vi "ParseCronExpression.vi"(8 "error in (no error)":errorcluster, 9 "values end":u32=59, 10 "values start":u32, 11 "expression":string="2, 45, 2-9,* /15") -> (0 "error out":errorcluster, 3 "comparisons":T1[](array[typedef]))   [LabVIEW 2017, in "CronScheduler.lvlib"]
uses:
  <vilib>/addons/InsightCM/Utilities/CronScheduler/CronScheduler.lvlib
  <vilib>/addons/InsightCM/Utilities/CronScheduler/controls/Compare.ctl
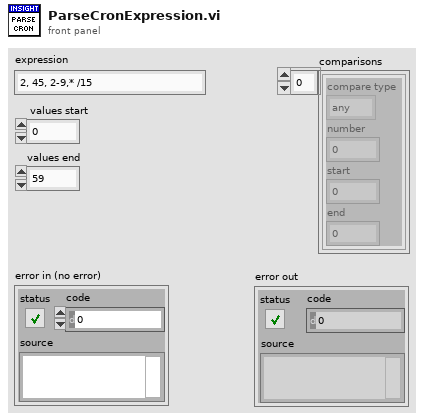
[diagram p1: front panel]
types:
  T1 = typedef "CronScheduler.lvlib/Compare.ctl" = cluster{"compare type":enum16{"any", "number", "range"}, "number":u32, "start":u32, "end":u32}
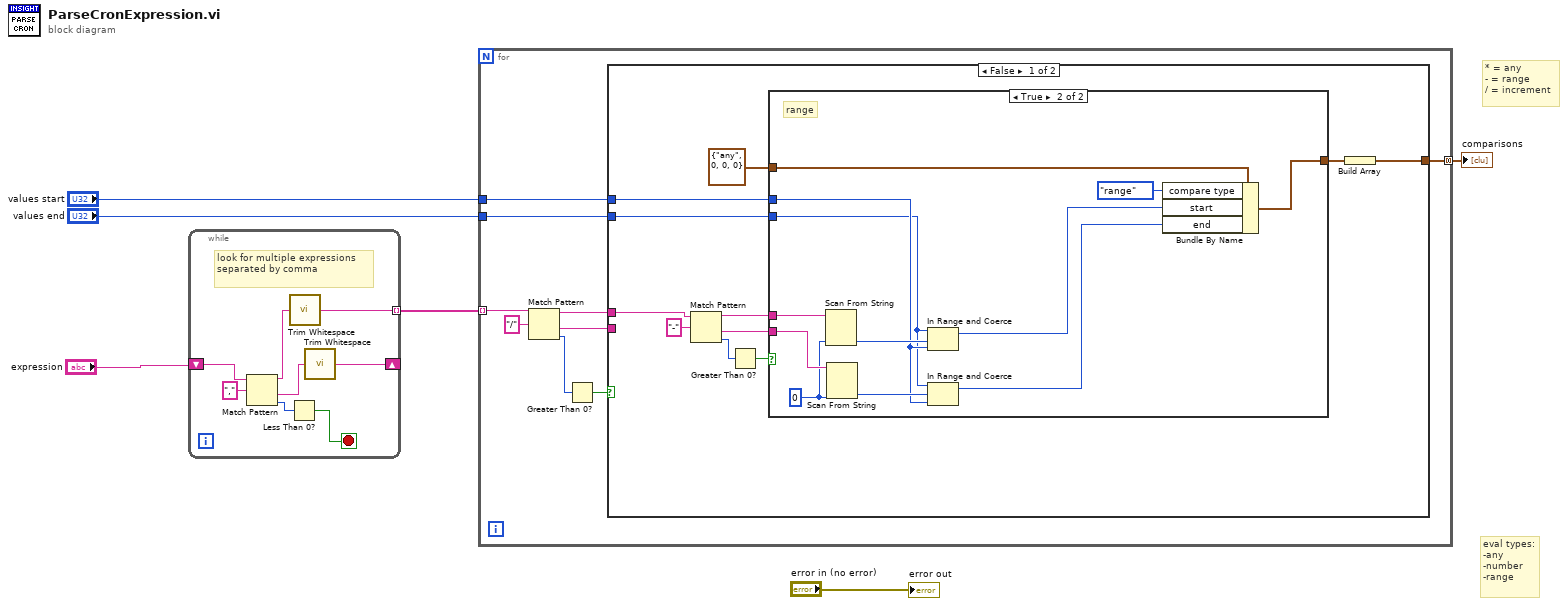
[diagram p0: block diagram]
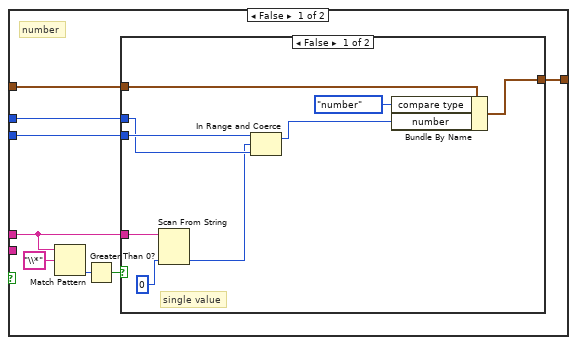
[diagram p2: hidden frame]
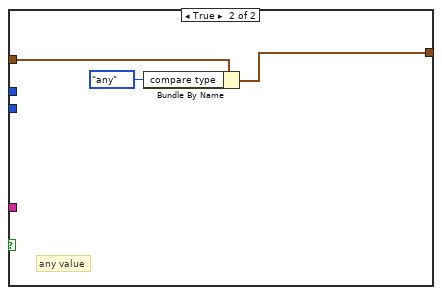
[diagram p3: hidden frame]
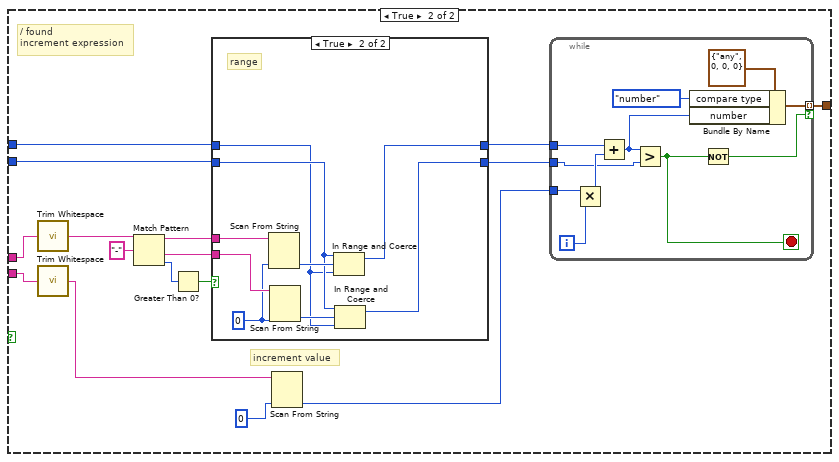
[diagram p4: hidden frame]
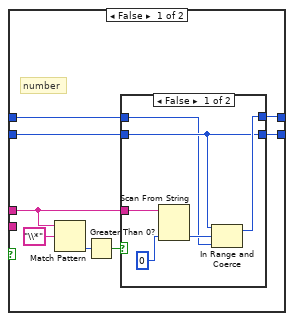
[diagram p5: hidden frame]
diagram:
  # "eval types:\n-any\n-number\n-range"
  # "* = any\n- = range\n/ = increment"
  n1 = while {
    shift-right: [w10] -> _
    shift-left: "expression" -> [w14]
    tunnel: [w11] -> w5 mode=indexing
    stop <- w8 stop-if-true
    # "look for multiple expressions separated by comma"
    n2 = Match Pattern(string=w14, regular expression=",") -> (before substring=w12:string, after substring=w9:string, offset past match=w13:i32)  [unwired: 1 in, 1 out]
    n3 = Less Than 0?(x=w13) -> (x < 0?=w8:bool)
    n4 = call <vilib>:"Trim Whitespace.vi"("string"=w12) -> ("trimmed string"=w11:string)  [unwired: 1 in]
    n5 = call <vilib>:"Trim Whitespace.vi"("string"=w9) -> ("trimmed string"=w10:string)  [unwired: 1 in]
  }
  n6 = for {
    tunnel: w5 -> [w23] mode=indexing
    tunnel: "values start" -> [w17]
    tunnel: "values end" -> [w16]
    tunnel: [w15] -> w2 mode=concatenating
    n7 = Match Pattern(string=w23, regular expression="/") -> (before substring=w19:string, after substring=w18:string, offset past match=w21:i32)  [unwired: 1 in, 1 out]
    n8 = Greater Than 0?(x=w21) -> (x > 0?=w20:bool)
    n9 = case shown="False" w20 {
      tunnel: w19 -> [w30 w82]
      tunnel: w18 -> [_ w81]
      tunnel: w17 -> [w25 w72]
      tunnel: w16 -> [w24 w71]
      tunnel: [w26 w67] -> w15
      frame False {
        n10 = Match Pattern(string=w30, regular expression="-") -> (before substring=w31:string, after substring=w32:string, offset past match=w34:i32)  [unwired: 1 in, 1 out]
        n11 = Greater Than 0?(x=w34) -> (x > 0?=w33:bool)
        n12 = case shown="True" w33 {
          tunnel: w32 -> [_ w65]
          tunnel: w31 -> [w42 w66]
          tunnel: T1 {"compare type"=enum."any", "number"=0, "start"=0, "end"=0} -> [w38 w63]
          tunnel: [w37 w62] -> w27
          tunnel: w25 -> [w36 w56]
          tunnel: w24 -> [w35 w55]
          frame False {
            # "number"
            n13 = Match Pattern(string=w42, regular expression="\\*") -> (offset past match=w40:i32)  [unwired: 1 in, 3 out]
            n14 = Greater Than 0?(x=w40) -> (x > 0?=w39:bool)
            n15 = case shown="False" w39 {
              tunnel: w42 -> [w50 _]
              tunnel: w38 -> [w49 w54]
              tunnel: [w48 w53] -> w37
              tunnel: w36 -> [w45 _]
              tunnel: w35 -> [w46 _]
              frame False {
                # "single value"
                n16 = Scan From String(input string=w50, default 1=u32 0) -> (output 1=w44:u32)  [unwired: 3 in, 3 out]
                n17 = In Range and Coerce(upper limit=w46, x=w44, lower limit=w45) -> (coerced(x)=w43:u32)  [unwired: 1 out]
                n18 = Bundle By Name(cluster=w49, "compare type"=enum16{"any", "number", "range"}."number", "number"=w43) -> (w48:T1)
              }
              frame True {
                # "any value"
                n19 = Bundle By Name(cluster=w54, "compare type"=enum16{"any", "number", "range"}."any") -> (w53:T1)
              }
            }
          }
          frame True {
            w64 = u32 0
            # "range"
            n20 = Scan From String(input string=w66, default 1=w64) -> (output 1=w60:u32)  [unwired: 3 in, 3 out]
            n21 = Scan From String(input string=w65, default 1=w64) -> (output 1=w58:u32)  [unwired: 3 in, 3 out]
            n22 = In Range and Coerce(upper limit=w55, x=w60, lower limit=w56) -> (coerced(x)=w59:u32)  [unwired: 1 out]
            n23 = In Range and Coerce(upper limit=w55, x=w58, lower limit=w56) -> (coerced(x)=w57:u32)  [unwired: 1 out]
            n24 = Bundle By Name(cluster=w63, "compare type"=enum16{"any", "number", "range"}."range", "start"=w59, "end"=w57) -> (w62:T1)
          }
        }
        n25 = Build Array(w27) -> (w26:T1[])
      }
      frame True {
        # "increment value"
        # "/ found\nincrement expression"
        n26 = call <vilib>:"Trim Whitespace.vi"("string"=w82) -> ("trimmed string"=w79:string)  [unwired: 1 in]
        n27 = call <vilib>:"Trim Whitespace.vi"("string"=w81) -> ("trimmed string"=w78:string)  [unwired: 1 in]
        n28 = Match Pattern(string=w79, regular expression="-") -> (before substring=w73:string, after substring=w74:string, offset past match=w76:i32)  [unwired: 1 in, 1 out]
        n29 = Greater Than 0?(x=w76) -> (x > 0?=w75:bool)
        n30 = case shown="True" w75 {
          tunnel: w74 -> [_ w117]
          tunnel: w73 -> [w101 w118]
          tunnel: w72 -> [w97 w110]
          tunnel: w71 -> [w96 w111]
          tunnel: [w95 w114] -> w70
          tunnel: [w94 w112] -> w68
          frame False {
            # "number"
            n31 = Match Pattern(string=w101, regular expression="\\*") -> (offset past match=w99:i32)  [unwired: 1 in, 3 out]
            n32 = Greater Than 0?(x=w99) -> (x > 0?=w98:bool)
            n33 = case shown="False" w98 {
              tunnel: w101 -> [w106 _]
              tunnel: w97 -> [w102 w109]
              tunnel: w96 -> [w103 w108]
              tunnel: [w104 w109] -> w95
              tunnel: [w103 w108] -> w94
              frame False {
                n34 = Scan From String(input string=w106, default 1=u32 0) -> (output 1=w105:u32)  [unwired: 3 in, 3 out]
                n35 = In Range and Coerce(upper limit=w103, x=w105, lower limit=w102) -> (coerced(x)=w104:u32)  [unwired: 1 out]
              }
              frame True {
                # "increment from start"
              }
            }
          }
          frame True {
            w116 = u32 0
            # "range"
            n36 = Scan From String(input string=w118, default 1=w116) -> (output 1=w115:u32)  [unwired: 3 in, 3 out]
            n37 = Scan From String(input string=w117, default 1=w116) -> (output 1=w113:u32)  [unwired: 3 in, 3 out]
            n38 = In Range and Coerce(upper limit=w111, x=w115, lower limit=w110) -> (coerced(x)=w114:u32)  [unwired: 1 out]
            n39 = In Range and Coerce(upper limit=w111, x=w113, lower limit=w110) -> (coerced(x)=w112:u32)  [unwired: 1 out]
          }
        }
        n40 = Scan From String(input string=w78, default 1=u32 0) -> (output 1=w69:u32)  [unwired: 3 in, 3 out]
        n41 = while {
          tunnel: w70 -> [w90]
          tunnel: w69 -> [w93]
          tunnel: w68 -> [w89]
          tunnel: [w86] -> w67 mode=indexing if=w85
          i -> [w92]
          stop <- w88 stop-if-true
          n42 = Multiply(x=w93, y=w92) -> (x*y=w91:u32)
          n43 = Add(x=w90, y=w91) -> (x+y=w84:u32)
          n44 = Greater?(x=w84, y=w89) -> (0:w88:bool)
          n45 = Bundle By Name(cluster=T1 {"compare type"=enum."any", "number"=0, "start"=0, "end"=0}, "compare type"=enum16{"any", "number", "range"}."number", "number"=w84) -> (w86:T1)
          n46 = Not(x=w88) -> (.not. x?=w85:bool)
        }
      }
    }
  }
  "comparisons" <- w2
  "error out" <- "error in (no error)"
